vi "MultiColumnList.vi"(0 "Stop Execution":bool, 5 "Combo Box":string(combo), 7 "error in":errorcluster) -> (4 "error out":errorcluster, 6 "Multicolumn Listbox":T1)   [LabVIEW 2020]
doc: "This is a multi column list box based Vi where a combo box is used to vary the values of the multi column list box"
uses:
  Typedefs/MultiColumnLists.ctl
panel:
  # "Click on any row or column to edit the items of \nmulti column list box"
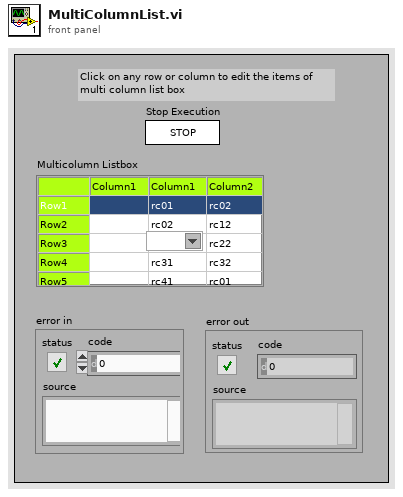
[diagram p1: front panel]
types:
  T1 = typedef "MultiColumnLists.ctl" = i32
  T2 = typedef "LVPoint32TypeDef.ctl" = cluster{"Horizontal":i32, "Vertical":i32}
  T3 = typedef "LVRowAndColumnTypeDef.ctl" = cluster{"Row":i32, "Column":i32}
  T4 = typedef "LVPositionTypeDef.ctl" = cluster{"Left":i32, "Top":i32}
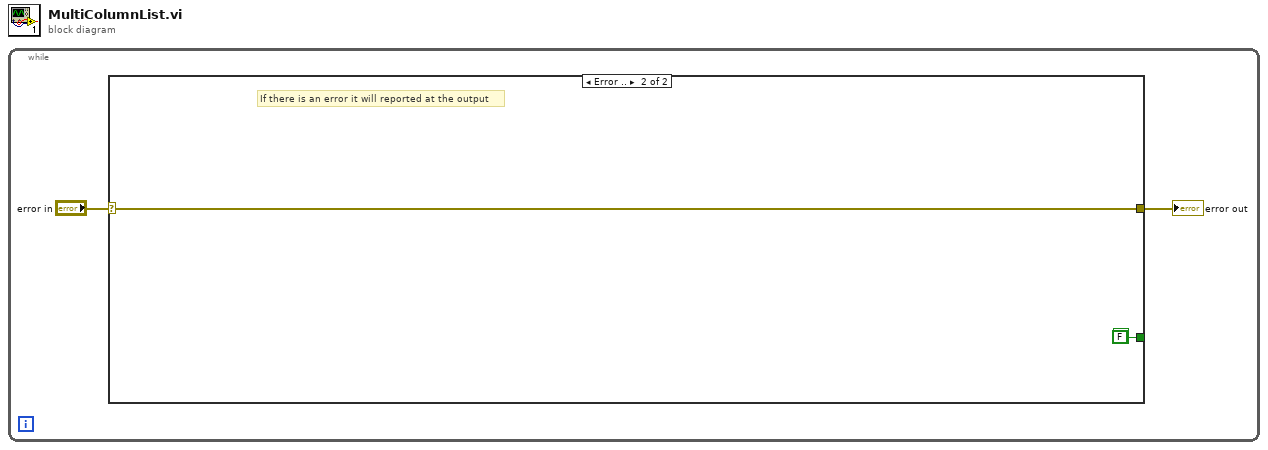
[diagram p0: block diagram]
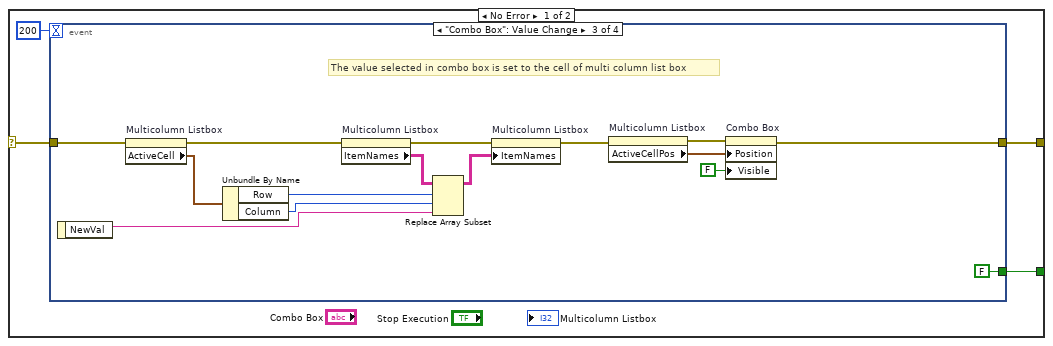
[diagram p2: hidden frame]
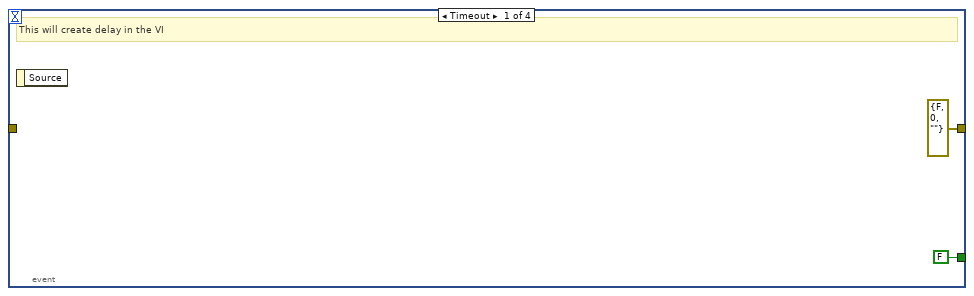
[diagram p3: hidden frame]
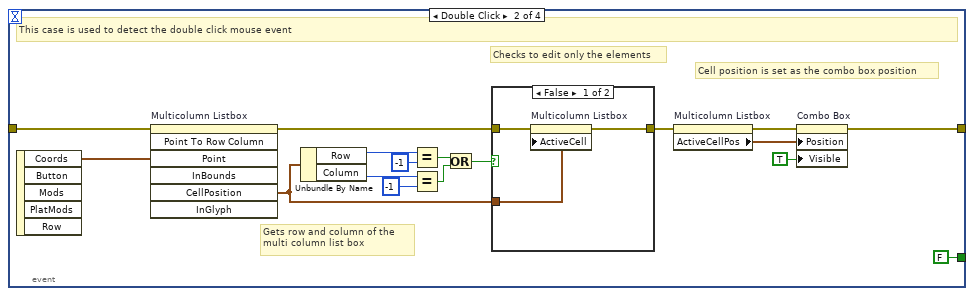
[diagram p4: hidden frame]
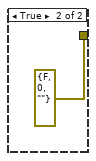
[diagram p5: hidden frame]
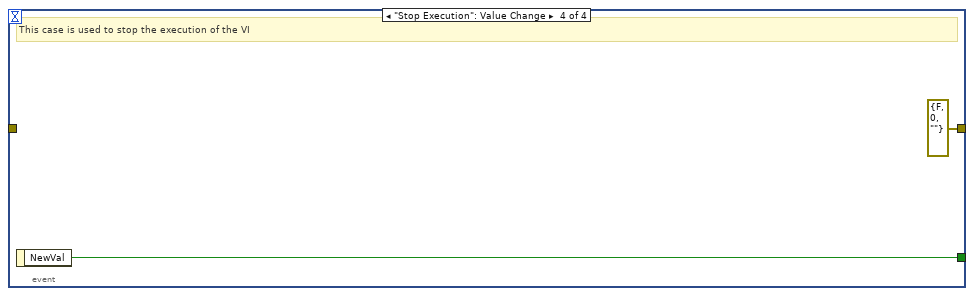
[diagram p6: hidden frame]
diagram:
  n1 = while {
    stop <- w3 stop-if-true
    n2 = case shown="Error .." "error in" {
      selector: "error in" -> [w4 w49]
      tunnel: [w7 FALSE ("NewVal")] -> w3
      tunnel: [w5 w49] -> w2
      frame No Error {
        n3 = event shown="[2] \"Combo Box\": Value Change" {
          selector: _ -> [_ _ _ _]
          dyn-events: _ -> [_ _ _ _]
          timeout: 200 -> [_ _ _ _]
          tunnel: [FALSE ("NewVal") FALSE ("NewVal") FALSE ("NewVal") w47] -> w7
          tunnel: [errorcluster {"status"=FALSE, "code"=0, "source"=""} ("error out") w11 w31 errorcluster {"status"=FALSE, "code"=0, "source"=""} ("error out")] -> w5
          tunnel: w4 -> [_ w10 w32 _]
          event Timeout {
            # "This will create delay in the VI"
            n4 = event-data() -> ()  [unwired: 1 in, 1 out]
          }
          event Double Click {
            # "Cell position is set as the combo box position"
            # "Gets row and column of the \nmulti column list box"
            # "Checks to edit only the elements"
            # "This case is used to detect the double click mouse event"
            n5 = event-data() -> ("Coords"=w26:T2)  [unwired: 1 in, 4 out]
            n6 = invoke on="Multicolumn Listbox" class="MCListbox (strict)" method="Point To Row Column"(error in=w10, "Point"=w26) -> (error out=w14:errorcluster, "CellPosition"=w18:T3)  [unwired: 5 in, 5 out]
            n7 = Unbundle By Name(w18) -> ("Row"=w25:i32, "Column"=w24:i32)
            n8 = Equal?(x=w25, y=-1) -> (x = y?=w21:bool)
            n9 = Equal?(x=w24, y=-1) -> (x = y?=w20:bool)
            n10 = Or(x=w21, y=w20) -> (x .or. y?=w19:bool)
            n11 = case shown="False" w19 {
              tunnel: w18 -> [w29 _]
              tunnel: [w28 errorcluster {"status"=FALSE, "code"=0, "source"=""} ("error in (no error)")] -> w15
              tunnel: w14 -> [w27 _]
              frame False {
                n12 = property on="Multicolumn Listbox" class="MCListbox (strict)"(error in=w27, "ActiveCell"=w29) -> (error out=w28:errorcluster)  [unwired: 1 in, 1 out]
              }
              frame True {
              }
            }
            n13 = property on="Multicolumn Listbox" class="MCListbox (strict)"(error in=w15) -> (error out=w13:errorcluster, "ActiveCellPos"=w17:T4)  [unwired: 1 in, 1 out]
            n14 = property on="Combo Box" class="CmbBox"(error in=w13, "Position"=w17, "Visible"=TRUE) -> (error out=w11:errorcluster)  [unwired: 1 in, 1 out]
          }
          event "Combo Box": Value Change {
            # "The value selected in combo box is set to the cell of multi column list box"
            n15 = event-data() -> ("NewVal"=w41:string)  [unwired: 1 in]
            n16 = property on="Multicolumn Listbox" class="MCListbox (strict)"(error in=w32) -> (error out=w38:errorcluster, "ActiveCell"=w45:T3)  [unwired: 1 in, 1 out]
            n17 = Unbundle By Name(w45) -> ("Row"=w43:i32, "Column"=w42:i32)
            n18 = property on="Multicolumn Listbox" class="MCListbox (strict)"(error in=w38) -> (error out=w39:errorcluster, "ItemNames"=w44:string[][])  [unwired: 1 in, 1 out]
            n19 = Replace Array Subset(array=w44, new element=w41, index (row)=w43, index (col)=w42) -> (w40:string[][])
            n20 = property on="Multicolumn Listbox" class="MCListbox (strict)"(error in=w39, "ItemNames"=w40) -> (error out=w33:errorcluster)  [unwired: 1 in, 1 out]
            n21 = property on="Multicolumn Listbox" class="MCListbox (strict)"(error in=w33) -> (error out=w37:errorcluster, "ActiveCellPos"=w36:T4)  [unwired: 1 in, 1 out]
            n22 = property on="Combo Box" class="CmbBox"(error in=w37, "Position"=w36, "Visible"=FALSE) -> (error out=w31:errorcluster)  [unwired: 1 in, 1 out]
          }
          event "Stop Execution": Value Change {
            # "This case is used to stop the execution of the VI"
            n23 = event-data() -> ("NewVal"=w47:bool)  [unwired: 1 in]
          }
        }
      }
      frame Error {
        # "If there is an error it will reported at the output"
      }
    }
    "error out" <- w2
  }
